vi "SOUR_CAT.vi"(0 "VISA IN":refnum<visa-resource-name>, 5 "error in":errorcluster, 7 "Channel":i32) -> (14 "VISA Out":refnum<visa-resource-name>, 16 "Data":string, 19 "error out":errorcluster)   [LabVIEW 2018, in "PNA-X.lvlib"]
doc: "SOURce<cnum>:CATalog? \n1823\n\n(Read-Write) Returns a list of valid port names that can be controlled. Some of these port names can \nNOT be accessed through the normal <port> argument used in many Source: commands. These string \nnames are used in the [src] argument. \nParameters \nExamples SOUR:CAT? \nsource:catalog \n'returns \n\"Port 1,Port 2,Port 3,Port 4,Port 1 Src2\" \nReturn Type Comma-separated list of strings. \nDefault Not applicable"
uses:
  PNA-X.lvlib
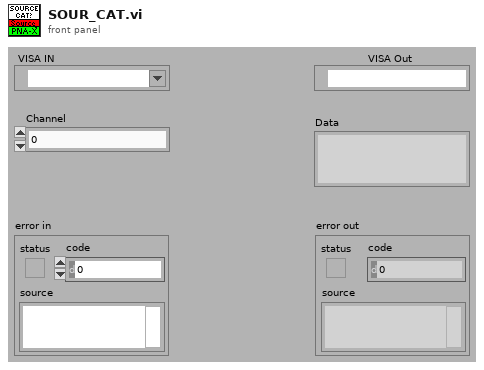
[diagram p1: front panel]
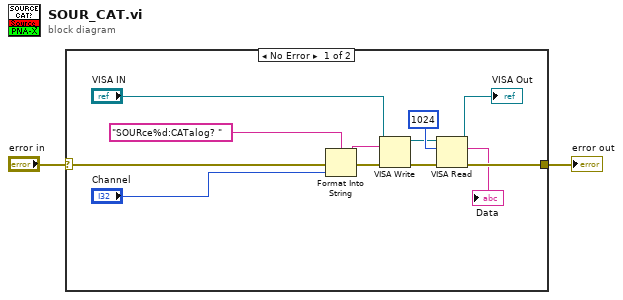
[diagram p0: block diagram]
diagram:
  n1 = case shown="No Error" "error in" {
    selector: "error in" -> [w14 w15]
    tunnel: [w6 w15] -> w1
    frame No Error {
      n2 = Format Into String(format string="SOURce%d:CATalog? " ("Cmdline"), error in=w14, "Channel") -> (resulting string=w12:string, error out=w13:errorcluster)  [unwired: 1 in]
      n3 = VISA Write(VISA resource name="VISA IN", write buffer=w12, error in (no error)=w13) -> (VISA resource name out=w7:refnum<visa-resource-name>, error out=w9:errorcluster)  [unwired: 1 out]
      n4 = VISA Read(VISA resource name=w7, byte count=1024, error in (no error)=w9) -> (VISA resource name out=→"VISA Out":refnum<visa-resource-name>, read buffer=→"Data":string, error out=w6:errorcluster)  [unwired: 1 out]
    }
    frame Error {
    }
  }
  "error out" <- w1
